vi "sub_download_waveforms.vi"(7 "Waveform base URI":string, 8 "error in":errorcluster, 10 "Filtered Waveforms in":T1[](array[typedef]), 11 "daq.io type in":T2={"daq.io ref"=refnum, "daq.io API Base"="", "Device Key"="", "Account ID"="", "online"=TRUE, "SSL"=FALSE}) -> (0 "error out":errorcluster, 1 "Waveform Labels out":string[](array[string]), 2 "Waveform Data out":waveform(dbl)[](array[waveform]), 3 "daq.io type out":T2={"daq.io ref"=refnum, "daq.io API Base"="", "Device Key"="", "Account ID"="", "online"=TRUE, "SSL"=FALSE}, 4 "time elapsed (ms)":u32)   [LabVIEW 2013, in "daqio minimal.lvlib"]
doc: "This VI downloads a specified Waveform document from daq.io."
uses:
  daqio minimal.lvlib
  _typedefs/daqio-Type.ctl
  <vilib>/httpClient/ClientHandle.ctl
  _typedefs/daqio-read-waveform-JSON-header-time.ctl
  _typedefs/daqio-read-waveform-JSON.ctl
  <vilib>/Easy HTTP Client/Easy HTTP.lvlib
  <vilib>/httpClient/LabVIEWHTTPClient.lvlib
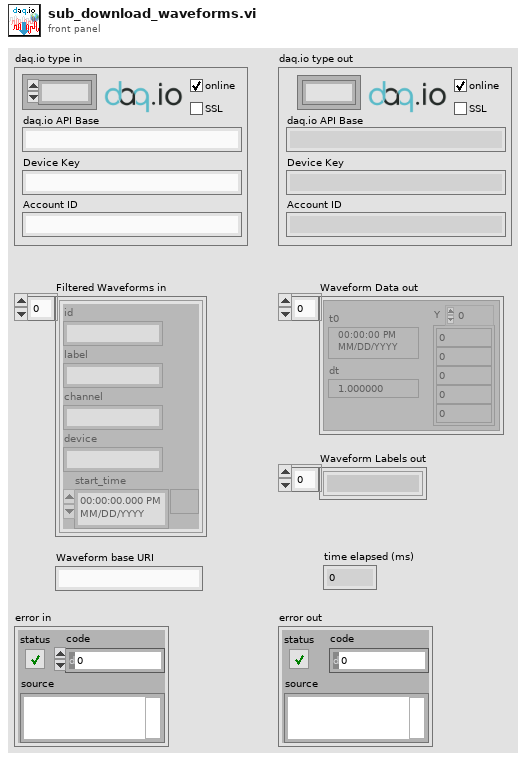
[diagram p1: front panel]
types:
  T1 = typedef "daqio minimal.lvlib/daqio-read-waveform-JSON-header-time.ctl" = cluster{"id":string, "label":string, "channel":string, "device":string, "start_time":timestamp}
  T2 = typedef "daqio minimal.lvlib/daqio-Type.ctl" = cluster{"daq.io ref":T3, "daq.io API Base":string, "Device Key":string, "Account ID":string, "online":bool, "SSL":bool}
  T3 = typedef "LabVIEWHTTPClient.lvlib/ClientHandle.ctl" = refnum<k1>
  T4 = typedef "daqio minimal.lvlib/daqio-read-waveform-JSON.ctl" = cluster{"start_time":string, "delta":dbl, "values":dbl[], "channel":string, "device":string, "label":string}
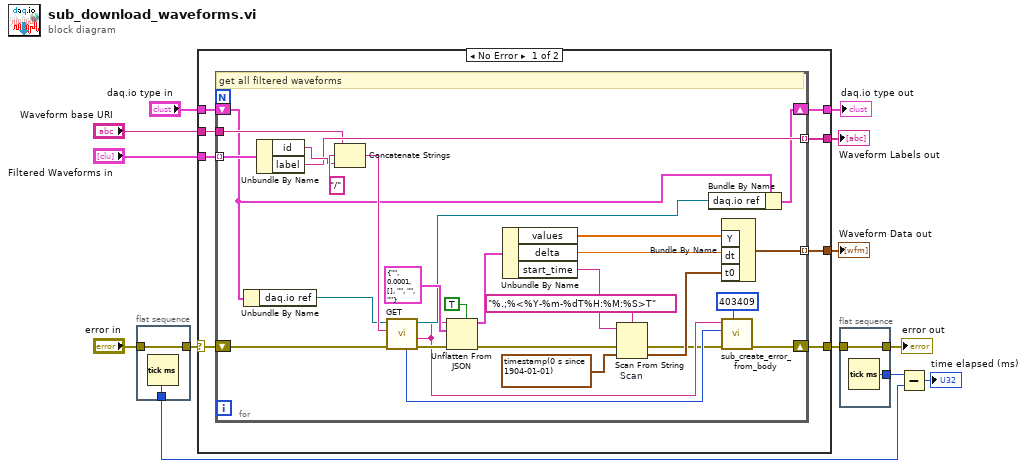
[diagram p0: block diagram]
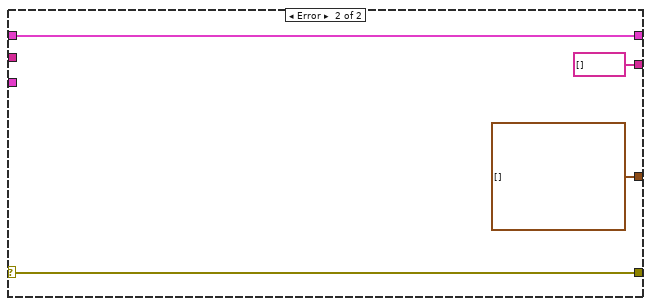
[diagram p2: hidden frame]
diagram:
  n1 = flat-sequence {
    tunnel: "error in" -> [w15]
    tunnel: [w15] -> w6
    tunnel: [w14] -> w2
    frame #0 {
      n2 = Tick Count (ms)() -> (millisecond timer value=w14:u32)
    }
  }
  n3 = case shown="No Error" w6 {
    selector: w6 -> [w16 w55]
    tunnel: [w23 w55] -> w5
    tunnel: [w22 w52] -> w13
    tunnel: "daq.io type in" -> [w21 w52]
    tunnel: "Filtered Waveforms in" -> [w20 _]
    tunnel: "Waveform base URI" -> [w19 _]
    tunnel: [w18 string[] []] -> w9
    tunnel: [w17 waveform(dbl)[] []] -> w8
    frame No Error {
      n4 = for {
        shift-right: [w24] -> w23
        shift-left: w16 -> [w45]
        tunnel: [w36] -> w17 mode=indexing
        tunnel: [w35] -> w18 mode=indexing
        shift-right: [w30] -> w22
        shift-left: w21 -> [w31]
        tunnel: w19 -> [w34]
        tunnel: w20 -> [w33] mode=indexing
        # "get all filtered waveforms"
        n5 = Unbundle By Name(w31) -> ("daq.io ref"=w32:T3)
        n6 = Unbundle By Name(w33) -> ("id"=w50:string, "label"=w35:string)
        n7 = Concatenate Strings(w34, "/" ("string"), w50) -> (w49:string)
        n8 = call <vilib>:"GET.vi"("error in (no error)"=w45, "url"=w49, "client handle"=w32) -> ("error out"=w47:errorcluster, "body"=w26:string, "client handle out"=w29:T3, "HTTP Response Code"=w27:i32)  [unwired: 4 in, 1 out]
        n9 = Unflatten From JSON(enable LabVIEW extensions? (T)=TRUE, JSON string=w26, type and defaults=T4 {"start_time"="", "delta"=0.0001, "values"=[], "channel"="", "device"="", "label"=""} ("Waveform"), error in (no error)=w47) -> (value=w44:T4, error out=w40:errorcluster)  [unwired: 3 in]
        n10 = Unbundle By Name(w44) -> ("values"=w39:dbl[], "delta"=w38:dbl, "start_time"=w43:string)
        n11 = Scan From String "Scan"(format string="%.;%<%Y-%m-%dT%H:%M:%S>T" ("input string"), input string=w43, error in=w40, default 1=timestamp(0 s since 1904-01-01) ("default value 1")) -> (error out=w25:errorcluster, output 1=w37:timestamp)  [unwired: 1 in, 2 out]
        n12 = Bundle By Name(cluster=w31, "daq.io ref"=w29) -> (w30:T2)
        n13 = Bundle By Name("Y"=w39, "dt"=w38, "t0"=w37) -> (w36:waveform(dbl))  [unwired: 1 in]
        n14 = call "sub_create_error_from_body.vi"("error code"=403409, "error in (no error)"=w25, "http code"=w27, "body"=w26) -> ("error out"=w24:errorcluster)  [unwired: 7 in]
      }
    }
    frame Error {
    }
  }
  "daq.io type out" <- w13
  "Waveform Labels out" <- w9
  "Waveform Data out" <- w8
  n15 = flat-sequence {
    tunnel: w5 -> [w57]
    tunnel: [w57] -> w4
    tunnel: [w56] -> w3
    frame #0 {
      n16 = Tick Count (ms)() -> (millisecond timer value=w56:u32)
    }
  }
  n17 = Subtract(x=w3, y=w2) -> (x-y=→"time elapsed (ms)":u32)
  "error out" <- w4
